vi "Enqueue Message (Single).vi"(8 "Error In":errorcluster, 9 "Message Position":T2=enum."Back", 10 "Data":variant, 11 "State Machine Message":T1) -> (0 "Error Out":errorcluster)   [LabVIEW 2023, in "QSM - Security.lvlib"]
doc: "This VI enqueues a message in the message queue at the specified position for the Queued State Machine template."
uses:
  QSM - Security.lvlib
  Controls/Message Queue Element Position.ctl
  Controls/State Machine Message.ctl
  Controls/Message Queue Reference Functional Global Variable Operation.ctl
  Controls/Message Queue Element.ctl
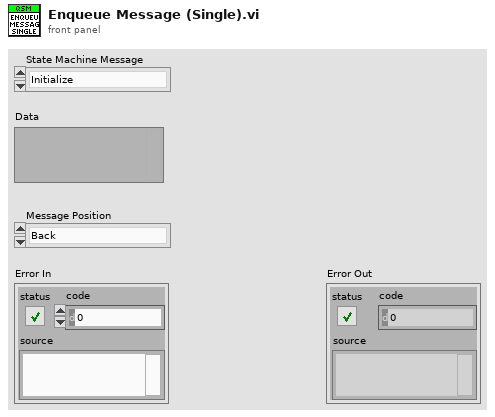
[diagram p1: front panel]
types:
  T1 = typedef "QSM - Security.lvlib/State Machine Message.ctl" = enum16{"Initialize", "Handle Error", "Exit"}
  T2 = typedef "QSM - Security.lvlib/Message Queue Element Position.ctl" = enum16{"Front", "Back"}
  T3 = typedef "QSM - Security.lvlib/Message Queue Element.ctl" = cluster{"State Machine Message":T1, "Data":variant}
  T4 = typedef "QSM - Security.lvlib/Message Queue Reference Functional Global Variable Operation.ctl" = enum16{"Set", "Get"}
  T5 = typedef "QSM - Library.lvlib/Message Queue Reference.ctl" = refnum<queue>
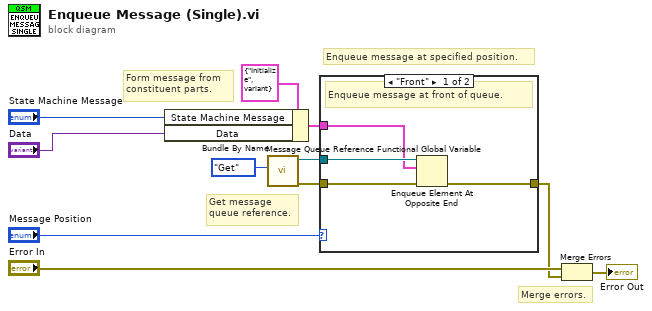
[diagram p0: block diagram]
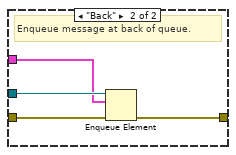
[diagram p2: hidden frame]
diagram:
  # "Merge errors."
  # "Form message from\nconstituent parts."
  # "Get message\nqueue reference."
  # "Enqueue message at specified position."
  n1 = Bundle By Name(cluster=T3 {"State Machine Message"=enum."Initialize", "Data"=variant} ("Message Queue Element"), "State Machine Message"="State Machine Message", "Data"="Data") -> (w6:T3)
  n2 = call "Message Queue Reference Functional Global Variable.vi"("Operation"=Message_Queue_Reference_Functional_Global_Variable_Operation."Get") -> ("Error Out"=w10:errorcluster, "Message Queue Reference Out"=w9:T5)  [unwired: 9 in]
  n3 = case shown="\"Front\"" "Message Position" {
    tunnel: [w15 w19] -> w2
    tunnel: w9 -> [w14 w18]
    tunnel: w6 -> [w13 w17]
    tunnel: w10 -> [w12 w16]
    frame "Front" {
      # "Enqueue message at front of queue."
      n4 = Enqueue Element At Opposite End(queue=w14, element=w13, error in (no error)=w12) -> (error out=w15:errorcluster)  [unwired: 1 in, 2 out]
    }
    frame "Back" {
      # "Enqueue message at back of queue."
      n5 = Enqueue Element(queue=w18, element=w17, error in (no error)=w16) -> (error out=w19:errorcluster)  [unwired: 1 in, 2 out]
    }
  }
  n6 = Merge Errors("Error In", w2) -> (→"Error Out":errorcluster)
